vi "CountingFPGA.vi"() -> ()   [LabVIEW 2016]
uses:
  <vilib>/rvi/Emulation/niFpgaGetClockAttributes.vi
  <vilib>/rvi/Emulation/niFpgaSctlEmulationGetInTimedLoop.vi
  <vilib>/rvi/Emulation/niFpgaEmulationReportErrorSimple.vi
  <vilib>/rvi/Emulation/niFpgaProcessEmulError.vi
  <vilib>/rvi/eio/common/nirviEmuTemplateMethod_errors.vi
  <vilib>/rvi/Emulation/niFpgaCriticalErrorInLSC.vi
  <vilib>/eio/EIONode/EIONode.xnode
panel:
  out "vVL":sgl
  out "vHR":sgl
  out "vHL":sgl
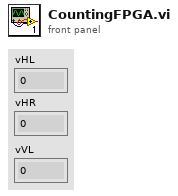
[diagram p1: front panel]
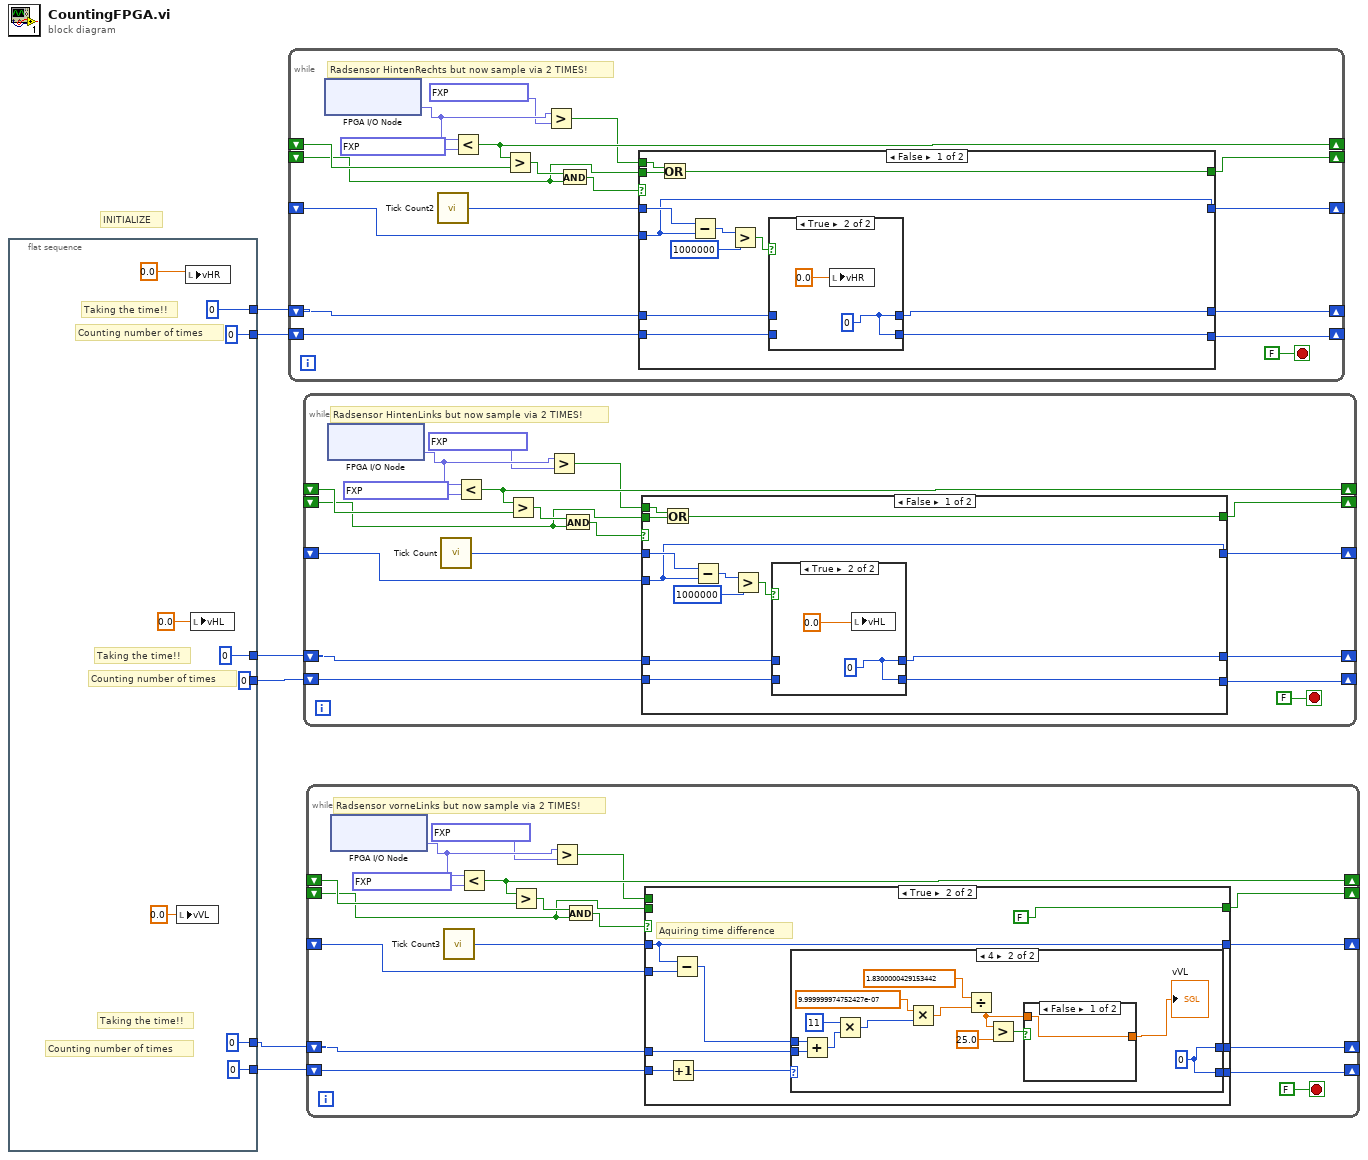
[diagram p0: block diagram]
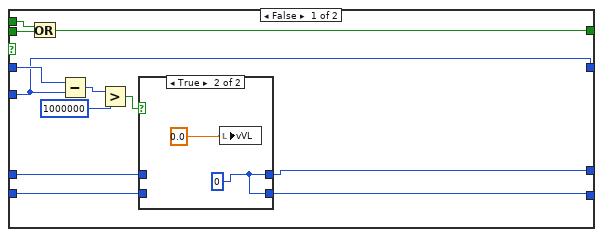
[diagram p2: hidden frame]
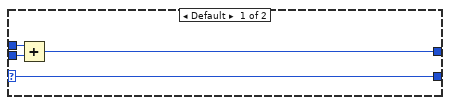
[diagram p4: hidden frame]
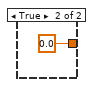
[diagram p5: hidden frame]
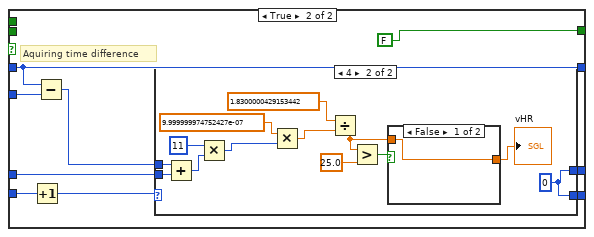
[diagram p7: hidden frame]
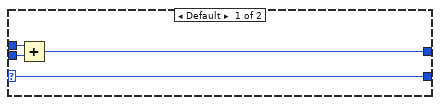
[diagram p8: hidden frame]
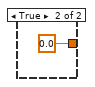
[diagram p9: hidden frame]
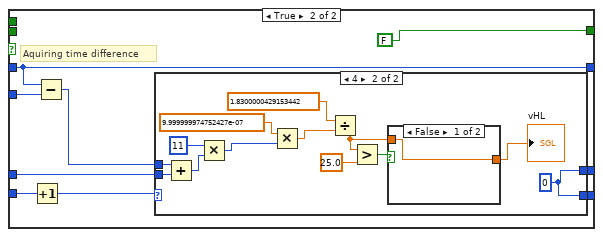
[diagram p11: hidden frame]
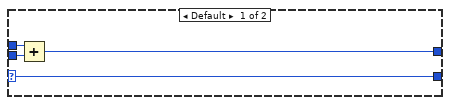
[diagram p12: hidden frame]
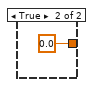
[diagram p13: hidden frame]
diagram:
  # "INITIALIZE"
  n1 = flat-sequence {
    tunnel: [i16 0] -> w6
    tunnel: [i16 0] -> w5
    tunnel: [i16 0] -> w4
    tunnel: [i16 0] -> w3
    tunnel: [i16 0] -> w2
    tunnel: [i16 0] -> w1
    frame #0 {
      # "Counting number of times"
      # "Taking the time!!"
      # "Taking the time!!"
      # "Counting number of times"
      # "Taking the time!!"
      # "Counting number of times"
      n2 = local write "vVL"(sgl 0.0 ("vVL")) -> ()
      n3 = local write "vHR"(sgl 0.0) -> ()
      n4 = local write "vHL"(sgl 0.0) -> ()
    }
  }
  n5 = while {
    shift-right: [w32] -> _
    shift-left: _ -> [w31]
    shift-right: [w29] -> _
    shift-left: _ -> [w28]
    shift-right: [w27] -> _
    shift-left: w3 -> [w26]
    shift-right: [w25] -> _
    shift-left: w4 -> [w24]
    shift-right: [w19] -> _
    shift-left: _ -> [w20]
    stop <- FALSE stop-if-true
    # "Radsensor HintenRechts but now sample via 2 TIMES!"
    n6 = xnode "FPGA I/O Node"() -> ("Mod2/AI0"=w18:fxp<+,18,3>)  [unwired: 1 in, 1 out]
    n7 = call "Tick Count2"() -> ("Tick Count(uSec)"=w30:u32)
    n8 = Less?(x=w18, y=fxp<+,18,3> 0.024993896484375) -> (x < y?=w32:bool)
    n9 = Greater?(x=w32, y=w31) -> (0:w23:bool)
    n10 = Greater?(x=w18, y=fxp<+,18,3> 0.32501220703125) -> (0:w21:bool)
    n11 = And(x=w23, y=w20) -> (x .and. y?=w22:bool)
    n12 = case shown="False" w22 {
      tunnel: w30 -> [w42 w58]
      tunnel: [w41 w58] -> w29
      tunnel: w28 -> [w41 w57]
      tunnel: w26 -> [w35 w56]
      tunnel: [w34 w54] -> w27
      tunnel: w24 -> [w37 w53]
      tunnel: [w36 w51] -> w25
      tunnel: w21 -> [w45 _]
      tunnel: w20 -> [w44 _]
      tunnel: [w43 FALSE] -> w19
      frame False {
        n13 = Or(x=w45, y=w44) -> (x .or. y?=w43:bool)
        n14 = Subtract(x=w42, y=w41) -> (x-y=w39:u32)
        n15 = Greater?(x=w39, y=u32 1000000) -> (0:w40:bool)
        n16 = case shown="True" w40 {
          tunnel: w37 -> [w47 _]
          tunnel: [w47 w49] -> w36
          tunnel: w35 -> [w46 _]
          tunnel: [w46 w49] -> w34
          frame False {
          }
          frame True {
            w49 = 0
            n17 = local write "vHR"(sgl 0.0) -> ()
          }
        }
      }
      frame True {
        # "Aquiring time difference"
        n18 = Increment(x=w56) -> (x+1=w55:i32)
        n19 = Subtract(x=w58, y=w57) -> (x-y=w52:u32)
        n20 = case shown="4" w55 {
          selector: w55 -> [w62 _]
          tunnel: [w62 w75] -> w54
          tunnel: w53 -> [w61 w74]
          tunnel: w52 -> [w60 w73]
          tunnel: [w59 w75] -> w51
          frame Default {
            n21 = Add(x=w60, y=w61) -> (x+y=w59:u32)
          }
          frame 4 {
            w75 = i16 0
            n22 = Add(x=w73, y=w74) -> (x+y=w72:u32)
            n23 = Multiply(x=u32 11, y=w72) -> (x*y=w69:u32)
            n24 = Multiply(x=sgl 1e-06, y=w69) -> (x*y=w67:sgl)
            n25 = Divide(x=sgl 1.83, y=w67) -> (x/y=w65:sgl)
            n26 = Greater?(x=w65, y=sgl 25.0) -> (0:w64:bool)
            n27 = case shown="False" w64 {
              tunnel: w65 -> [w76 _]
              tunnel: [w76 sgl 0.0] -> w63
              frame False {
              }
              frame True {
              }
            }
            "vHR" <- w63
          }
        }
      }
    }
  }
  n28 = while {
    shift-right: [w94] -> _
    shift-left: _ -> [w93]
    shift-right: [w91] -> _
    shift-left: _ -> [w90]
    shift-right: [w89] -> _
    shift-left: w5 -> [w88]
    shift-right: [w87] -> _
    shift-left: w6 -> [w86]
    shift-right: [w81] -> _
    shift-left: _ -> [w82]
    stop <- FALSE stop-if-true
    # "Radsensor HintenLinks but now sample via 2 TIMES!"
    n29 = xnode "FPGA I/O Node"() -> ("Mod2/AI1"=w80:fxp<+,18,3>)  [unwired: 1 in, 1 out]
    n30 = call "Tick Count"() -> ("Tick Count(uSec)"=w92:u32)
    n31 = Less?(x=w80, y=fxp<+,18,3> 0.024993896484375) -> (x < y?=w94:bool)
    n32 = Greater?(x=w94, y=w93) -> (0:w85:bool)
    n33 = Greater?(x=w80, y=fxp<+,18,3> 0.29998779296875) -> (0:w83:bool)
    n34 = And(x=w85, y=w82) -> (x .and. y?=w84:bool)
    n35 = case shown="False" w84 {
      tunnel: w92 -> [w104 w120]
      tunnel: [w103 w120] -> w91
      tunnel: w90 -> [w103 w119]
      tunnel: w88 -> [w97 w118]
      tunnel: [w96 w116] -> w89
      tunnel: w86 -> [w99 w115]
      tunnel: [w98 w113] -> w87
      tunnel: w83 -> [w107 _]
      tunnel: w82 -> [w106 _]
      tunnel: [w105 FALSE] -> w81
      frame False {
        n36 = Or(x=w107, y=w106) -> (x .or. y?=w105:bool)
        n37 = Subtract(x=w104, y=w103) -> (x-y=w101:u32)
        n38 = Greater?(x=w101, y=u32 1000000) -> (0:w102:bool)
        n39 = case shown="True" w102 {
          tunnel: w99 -> [w109 _]
          tunnel: [w109 w111] -> w98
          tunnel: w97 -> [w108 _]
          tunnel: [w108 w111] -> w96
          frame False {
          }
          frame True {
            w111 = 0
            n40 = local write "vHL"(sgl 0.0) -> ()
          }
        }
      }
      frame True {
        # "Aquiring time difference"
        n41 = Increment(x=w118) -> (x+1=w117:i32)
        n42 = Subtract(x=w120, y=w119) -> (x-y=w114:u32)
        n43 = case shown="4" w117 {
          selector: w117 -> [w124 _]
          tunnel: [w124 w137] -> w116
          tunnel: w115 -> [w123 w136]
          tunnel: w114 -> [w122 w135]
          tunnel: [w121 w137] -> w113
          frame Default {
            n44 = Add(x=w122, y=w123) -> (x+y=w121:u32)
          }
          frame 4 {
            w137 = i16 0
            n45 = Add(x=w135, y=w136) -> (x+y=w134:u32)
            n46 = Multiply(x=u32 11, y=w134) -> (x*y=w131:u32)
            n47 = Multiply(x=sgl 1e-06, y=w131) -> (x*y=w129:sgl)
            n48 = Divide(x=sgl 1.83, y=w129) -> (x/y=w127:sgl)
            n49 = Greater?(x=w127, y=sgl 25.0) -> (0:w126:bool)
            n50 = case shown="False" w126 {
              tunnel: w127 -> [w138 _]
              tunnel: [w138 sgl 0.0] -> w125
              frame False {
              }
              frame True {
              }
            }
            "vHL" <- w125
          }
        }
      }
    }
  }
  n51 = while {
    shift-right: [w156] -> _
    shift-left: _ -> [w155]
    shift-right: [w153] -> _
    shift-left: _ -> [w152]
    shift-right: [w151] -> _
    shift-left: w2 -> [w150]
    shift-right: [w149] -> _
    shift-left: w1 -> [w148]
    shift-right: [w143] -> _
    shift-left: _ -> [w144]
    stop <- FALSE stop-if-true
    # "Radsensor vorneLinks but now sample via 2 TIMES!"
    n52 = xnode "FPGA I/O Node"() -> ("Mod2/AI2"=w142:fxp<+,18,3>)  [unwired: 1 in, 1 out]
    n53 = call "Tick Count3"() -> ("Tick Count(uSec)"=w154:u32)
    n54 = Less?(x=w142, y=fxp<+,18,3> 0.00799560546875) -> (x < y?=w156:bool)
    n55 = Greater?(x=w156, y=w155) -> (0:w147:bool)
    n56 = Greater?(x=w142, y=fxp<+,18,3> 0.05999755859375) -> (0:w145:bool)
    n57 = And(x=w147, y=w144) -> (x .and. y?=w146:bool)
    n58 = case shown="True" w146 {
      tunnel: w154 -> [w166 w182]
      tunnel: [w165 w182] -> w153
      tunnel: w152 -> [w165 w181]
      tunnel: w150 -> [w159 w180]
      tunnel: [w158 w178] -> w151
      tunnel: w148 -> [w161 w177]
      tunnel: [w160 w175] -> w149
      tunnel: w145 -> [w169 _]
      tunnel: w144 -> [w168 _]
      tunnel: [w167 FALSE] -> w143
      frame False {
        n59 = Or(x=w169, y=w168) -> (x .or. y?=w167:bool)
        n60 = Subtract(x=w166, y=w165) -> (x-y=w163:u32)
        n61 = Greater?(x=w163, y=u32 1000000) -> (0:w164:bool)
        n62 = case shown="True" w164 {
          tunnel: w161 -> [w171 _]
          tunnel: [w171 w173] -> w160
          tunnel: w159 -> [w170 _]
          tunnel: [w170 w173] -> w158
          frame False {
          }
          frame True {
            w173 = 0
            n63 = local write "vVL"(sgl 0.0) -> ()
          }
        }
      }
      frame True {
        # "Aquiring time difference"
        n64 = Increment(x=w180) -> (x+1=w179:i32)
        n65 = Subtract(x=w182, y=w181) -> (x-y=w176:u32)
        n66 = case shown="4" w179 {
          selector: w179 -> [w186 _]
          tunnel: [w186 w199] -> w178
          tunnel: w177 -> [w185 w198]
          tunnel: w176 -> [w184 w197]
          tunnel: [w183 w199] -> w175
          frame Default {
            n67 = Add(x=w184, y=w185) -> (x+y=w183:u32)
          }
          frame 4 {
            w199 = i16 0
            n68 = Add(x=w197, y=w198) -> (x+y=w196:u32)
            n69 = Multiply(x=u32 11, y=w196) -> (x*y=w193:u32)
            n70 = Multiply(x=sgl 1e-06, y=w193) -> (x*y=w191:sgl)
            n71 = Divide(x=sgl 1.83, y=w191) -> (x/y=w189:sgl)
            n72 = Greater?(x=w189, y=sgl 25.0) -> (0:w188:bool)
            n73 = case shown="False" w188 {
              tunnel: w189 -> [w200 _]
              tunnel: [w200 sgl 0.0] -> w187
              frame False {
              }
              frame True {
              }
            }
            "vVL" <- w187
          }
        }
      }
    }
  }
